vi "projekt 2.vi"() -> ()   [LabVIEW 2017]
panel:
  in  "index":i32
  out "size(s)":i32
  out "element":dbl
  out "Array":dbl[](array[slide]) scale=0.0..10.0
  in  "Array":dbl[](array[numeric])
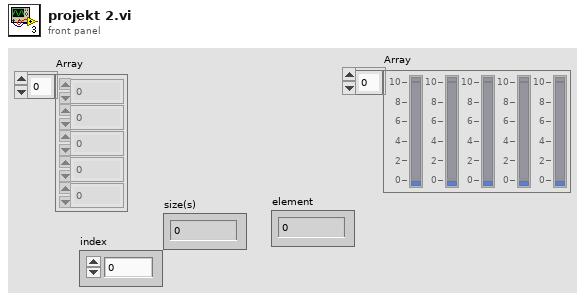
[diagram p1: front panel]
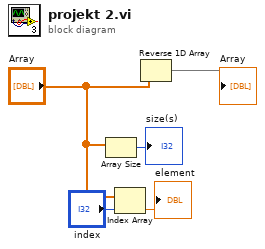
[diagram p0: block diagram]
diagram:
  n1 = Array Size(array="Array") -> (size(s)=→"size(s)":i32)
  n2 = Index Array(array="Array", index="index") -> (element=→"element":dbl)
  n3 = Reverse 1D Array(array="Array") -> (reversed array=→"Array":dbl[])
